vi "AlliGator Batch Dataset Export Window.vi"() -> ()   [LabVIEW 2021, in "AlliGator Files.lvlib"]
doc: "GUI for batch .ptu datasets export to HDF5 files or folders of TIFF images."
uses:
  AlliGator Files.lvlib
  Scripts/AlliGator Data Load & Process Options.ctl
  Scripts/AlliGator Data Information.ctl
  Settings/AlliGator Background Subtraction Parameters.ctl
  Settings/AlliGator Define Gates to.ctl
  Settings/AlliGator Gates to Keep.ctl
  Settings/AlliGator Gate Arithmetic.ctl
  Scripts/AlliGator Source Image Settings.ctl
  Settings/AlliGator Low Count Pixels Rejection Options.ctl
  Settings/AlliGator High Count Pixels Rejection Options.ctl
  Settings/AlliGator Image Smoothing Options.ctl
  Arrays/Kernel Type.ctl
  Arrays/Smoothing Algorithm.ctl
  Source Image/AlliGator Image Binning Options.ctl
  Decay Analysis/Decay Preprocessing/AlliGator Decay Preprocessing Options.ctl
  Decay Analysis/Decay Preprocessing/AlliGator Background Subtraction Parameters.ctl
  Decay Analysis/Decay Preprocessing/AlliGator Baseline Subtraction Method.ctl
  Decay Analysis/Decay Preprocessing/AlliGator Decay Preprocessing Parameters.ctl
  Graphs/XY Graph/XY Graph Plot Shift Parameters.ctl
  Graphs/XY Graph/XY Graph Plot Shift Method.ctl
  Globals, Variables, Constants/AlliGator Variables List.ctl
  AlliGator Batch File Conversion Item.ctl
  AlliGator TIFF Series Options.ctl
  AlliGator Saved TIFF Image Type.ctl
  835454da-008c-4cc5-9e1e-46d3d2ae4ada.vi
  <userlib>/_OpenG.lib/array/array.llb/Filter 1D Array with Scalar (Boolean)__ogtk.vi
  <userlib>/_OpenG.lib/array/array.llb/Delete Elements from 1D Array (Variant)__ogtk.vi
  Variant/Variant to Data/Variant to Boolean.vi
  <vilib>/ErrorRing/Error Ring.xnode
  GUI/GUI.lvlib
  <userlib>/_OpenG.lib/array/array.llb/openg_array.lvlib
  Scripts/AlliGator Scripts.lvlib
  Settings/AlliGator Settings.lvlib
  Arrays/Arrays.lvlib
  Source Image/AlliGator Source Image.lvlib
  Decay Analysis/Decay Preprocessing/AlliGator Decay Preprocessing.lvlib
  Graphs/XY Graph/XY Graph Add-Ons.lvlib
  Notebook/Notebook.lvlib
  Rich Text Box/Rich Text Box.lvlib
  Strings/Strings.lvlib
  Globals, Variables, Constants/AlliGator Globals, Variables & Constants.lvlib
  Variant/Variant to Data/Variant to Data.lvlib
  Sound/Sound.lvlib
  Utilities/Utilities.lvlib
panel:
  out "Conversion Jobs":cluster{"File Path":path, "Exported":bool}[](array[cluster])
  out "Message":string
  out "Animated Busy Icon":bool=TRUE
  in  "Abort":bool
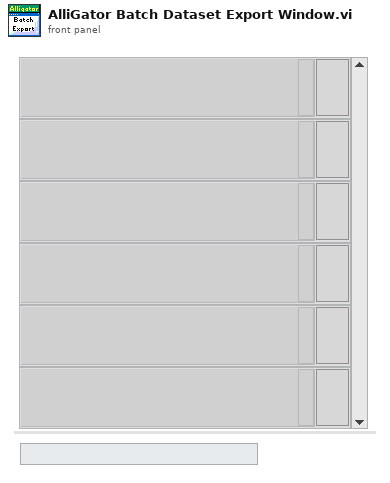
[diagram p1: front panel]
types:
  T1 = typedef "AlliGator Globals, Variables & Constants.lvlib/AlliGator Variables List.ctl" = enum16{"---- GUI ----", "GUI:Initialization Status", "GUI:State Indicators Refnum", "GUI:Original AlliGator Menu Items", "GUI:Current Action Loop State", "GUI:Script in progress", "GUI:Playback", "GUI:Loop Playback", "GUI:Search ROI Used", "GUI:Search ROI", "Decay Graph Max Legend Size", "Intensity Graph Max Legend Size", "Decay Statistics Graph Max Legend Size", "Phasor Graph Max Legend Size", "Phasor Ratio Graph Max Legend Size", "Lifetime Graph Max Legend Size", "---- Files ----", "Files:Export Dataset Frames as Individual Files", "Files:Show Batch Export Help Balloons", "Files:Frames in Dataset", "Files:ptu File Frame Start Indices", "Files:Current Frame in Dataset", "Files:Current Frame Timestamp", "Files:Dataset Loaded", "Files:Dataset Metadata", "Files:Dataset Channel", "Files:Dataset Data Description", "Files:Background Dataset Metadata", "Files:Background Dataset Channel", "Files:Background Dataset Data Description", "Files:Background File Subtraction", "Files:Background File Path", "Files:Background File Pile-up Correction", "Files:Background File Pixel Well Capacity", "Files:Background File Scaling Factor", "Files:Current Dataset Load Settings", "Files:Dataset Path", "Files:ICCD-specific Information", "Files:Macrotime Gate Separation", "------ Python Plugins ------", "Python Plugins:Information", "Python Plugins:Python Session", "Python Plugins:Valid Python Session?", "---- Source Image ----", "Source Image:ROIs", "Source Image:Current ROI", "Source Image:ROI Event Refnum", "X_Source Image Display Range", "X_Source Image Palette Information", "X_Type of Displayed Image", "X_Time Gate Slider", "Source Image:Palette List", "Source Image:Scale", "Source Image:ROI Overlay Color", "Source Image:Overlay to Erase", "Source Image:Is Displayed Image Accumulated", "Source Image:White Light Image Modified", "Source Image:Mask Image Modified", "---- Image Profile Window ----", "Image Profile:Window Event Refnum", "Image Profile:IntensityType", "Image Profile:Intensity Average Type", "Image Profile:Intensity-weighted SDV", "Image Profile:Box Profile Type", "Image Profile:Window Open", "Image Profile:Plotted Fit Parameter", "------ Phasor Graph -------", "Phasor Graph:Show Line", "---- Phasor Plot ---", "Phasor Plot:Parameters Changed", "Phasor Plot:FLI Dataset Modified since last Calculation", "Phasor Harmonics Data", "Selected Phasor Harmonics", "Phasor Harmonic Manager Event Refnum", "Phasor Plot:ROIs", "Phasor Plot:Current ROI", "Phasor Plot:ROI Event Refnum", "Phasor Plot:Image Reference Points", "Phasor Plot:Computed", "Phasor Plot:Palette Information", "Phasor Plot:Palette List", "Phasor Plot:Phasor Ratio Palette Information", "Phasor Plot:Phasor Ratio Palette List", "Phasor Plot:Image Scale", "Phasor Plot:Image Overlay to Erase", "Phasor Plot:Image Elements to Update", "Phasor Plot:Current Calculation Parameters", "Phasor Plot:Current Calibration Options", "Phasor Plot:Reset Cumulated Phasor Plot", "Phasor Plot:Reference 1", "Phasor Plot:Lifetime Reference 1", "Phasor Plot:Reference 1 Frequency", "Phasor Plot:Reference 2", "Phasor Plot:Lifetime Reference 2", "Phasor Plot:Reference 2 Frequency", "---- Decay Analysis ----", "Number of Selected Decays to Fit", "LS Fit Results", "LAR Fit Results", "BS Fit Results", "Last Decay Max - Min", "Best Fit Parameters", "Best Fit Parameter Names", "Actual Size X", "Actual Size Y", "Binning X", "Binning Y", "Actual # Gates", "Dataset Number", "Gates to...", "Gates Skipped", "Gates to keep", "Gate Step", "Gate Separation", "Reversed Gates", "Pile-up Correction", "Pixel Well Capacity", "Background Subtracted", "Background Subtraction Method", "Background Definition Range", "Background File (deprecated)", "Number of Dataset Accumulated", "Array of Accumulated Dataset Paths", "Do Averaged Datasets", "Destination File Path", "Process Plot Target", "Use 1/D as Phasor Frequency", "---- Decay Fit Parameter Map -----", "Decay Fit Parameter Map:Palette Information", "Decay Fit Parameter Map:Palette List", "---- Parameter Map ----", "Parameter Map:Palette Information", "Parameter Map:Palette List", "------- Local Decay Window ---------", "Local Decay Graph Window:Event Refnum", "Local Decay Graph Window:Use normalized IRF for convolution", "----- Miscellaneous ----", "Misc:Skippable Dialog Windows Status"}
  T2 = typedef "AlliGator Scripts.lvlib/AlliGator Data Load & Process Options.ctl" = cluster{"Data Information":T3, "Source Image Settings":T8, "Decay Preprocessing Options & Parameters":T15, "Clear Phasor Graph":bool}
  T3 = typedef "AlliGator Scripts.lvlib/AlliGator Data Information.ctl" = cluster{"Gates to Skip":T4, "# Gates":u32, "Gate Step":u32, "Gate Duration":dbl[unit], "Gate Separation":dbl[unit], "Pile-up Correction":bool, "Pixel Well Capacity":u32, "Define Gates to":T5, "Gates to Keep":T6, "Laser Period":dbl[unit], "SYNC Period":dbl[unit], "Channel Name":u16, "Channel Arithmetic":T7, "Background File Subtraction":bool, "Background Scaling Factor":dbl, "Background File":path, "Background Pile-up Correction":bool, "Background Pixel Well Capacity":u32, "Dataset Scaling Factor":dbl}
  T4 = typedef "AlliGator Settings.lvlib/AlliGator Background Subtraction Parameters.ctl" = cluster{"Start":u32, "End":u32}
  T5 = typedef "AlliGator Settings.lvlib/AlliGator Define Gates to.ctl" = enum32{"Skip", "Keep"}
  T6 = typedef "AlliGator Settings.lvlib/AlliGator Gates to Keep.ctl" = cluster{"First":u32, "Last":u32}
  T7 = typedef "AlliGator Settings.lvlib/AlliGator Gate Arithmetic.ctl" = enum16{"None", "INT-G2", "G2/INT*<INT>", "(1 - G2/INT)*<INT>"}
  T8 = typedef "AlliGator Scripts.lvlib/AlliGator Source Image Settings.ctl" = cluster{"Low Count Pixels Rejection Options":T9, "High Count Pixels Rejection Options":T10, "Peak Threshold":dbl, "Intensity Threshold":dbl, "Image Smoothing Options":T11, "Image Binning Options":T14}
  T9 = typedef "AlliGator Settings.lvlib/AlliGator Low Count Pixels Rejection Options.ctl" = cluster{"Background Low Threshold Factor":dbl, "Fixed Low Background Threshold":dbl, "Reject Low Count Pixels":bool, "Low Percentile":dbl}
  T10 = typedef "AlliGator Settings.lvlib/AlliGator High Count Pixels Rejection Options.ctl" = cluster{"Background High Threshold Factor":dbl, "Fixed High Background Threshold":dbl, "Reject High Count Pixels":bool, "High Percentile":dbl}
  T11 = typedef "AlliGator Settings.lvlib/AlliGator Image Smoothing Options.ctl" = cluster{"Use Image Smoothing":bool, "Kernel Type":T12, "Bin":i32, "Algorithm":T13}
  T12 = typedef "Arrays.lvlib/Kernel Type.ctl" = enum16{"Uniform", "Bilinear", "Gaussian"}
  T13 = typedef "Arrays.lvlib/Smoothing Algorithm.ctl" = enum16{"Rapid", "Thorough"}
  T14 = typedef "AlliGator Source Image.lvlib/AlliGator Image Binning Options.ctl" = cluster{"Use Image Binning":bool, "X Bin":i32, "Y Bin":i32}
  T15 = typedef "AlliGator Decay Preprocessing.lvlib/AlliGator Decay Preprocessing Options.ctl" = cluster{"Background Subtraction Parameters":T16, "Decay Preprocessing Parameters":T18, "Preprocessing Steps Order":string[]}
  T16 = typedef "AlliGator Decay Preprocessing.lvlib/AlliGator Background Subtraction Parameters.ctl" = cluster{"Background Definition Range":cluster{"Min Gate":dbl[unit], "Max Gate":dbl[unit]}, "Baseline Subtraction Method":T17, "Background Subtraction?":bool, "Background File":path, "Background Constant":dbl, "Background Scaling Factor":dbl, "Background Pile-up Correction":bool, "Background Pixel Well Capacity":u32}
  T17 = typedef "AlliGator Decay Preprocessing.lvlib/AlliGator Baseline Subtraction Method.ctl" = enum16{"Mean", "Min", "Square Gated Single-Exponential", "File", "Constant"}
  T18 = typedef "AlliGator Decay Preprocessing.lvlib/AlliGator Decay Preprocessing Parameters.ctl" = cluster{"Background Subtraction":bool, "Straighten Decay":bool, "Reverse Gates":bool, "1-Normalized Decay":bool, "Smoothen Decay":bool, "Smoothing Parameter":dbl, "Shift Decay":bool, "Decay Shift Parameters":T19, "Extrapolate Decay":bool, "Additional Points":u32, "Head Fraction":dbl, "Pixel-Normalize Decay":bool, "Use Periodicity":bool, "Use Cursors":bool, "Tail Fraction":dbl, "Use Decay Pre-Processing":bool, "Fold Decay":bool, "# Folds":u32, "[0-1]-Normalized Decay":bool}
  T19 = typedef "XY Graph Add-Ons.lvlib/XY Graph Plot Shift Parameters.ctl" = cluster{"Type":T20, "Shift":dbl[unit], "Threshold":dbl, "Rotate":bool}
  T20 = typedef "XY Graph Add-Ons.lvlib/XY Graph Plot Shift Method.ctl" = enum16{"Default", "CFD", "Threshold", "Cross-Correlation"}
  T21 = typedef "AlliGator Files.lvlib/AlliGator Batch File Conversion Item.ctl" = cluster{"File Path":path, "Saved":bool}
  T22 = typedef "AlliGator Files.lvlib/AlliGator Saved TIFF Image Type.ctl" = enum16{"Single Gate", "Sum of All Gates", "Phasor"}
  T23 = typedef "AlliGator Files.lvlib/AlliGator TIFF Series Options.ctl" = cluster{"Gate Image File Name":string, "File Number Format":string, "Start Index":u32, "Save Metadata File":bool, "Compress Image":bool}
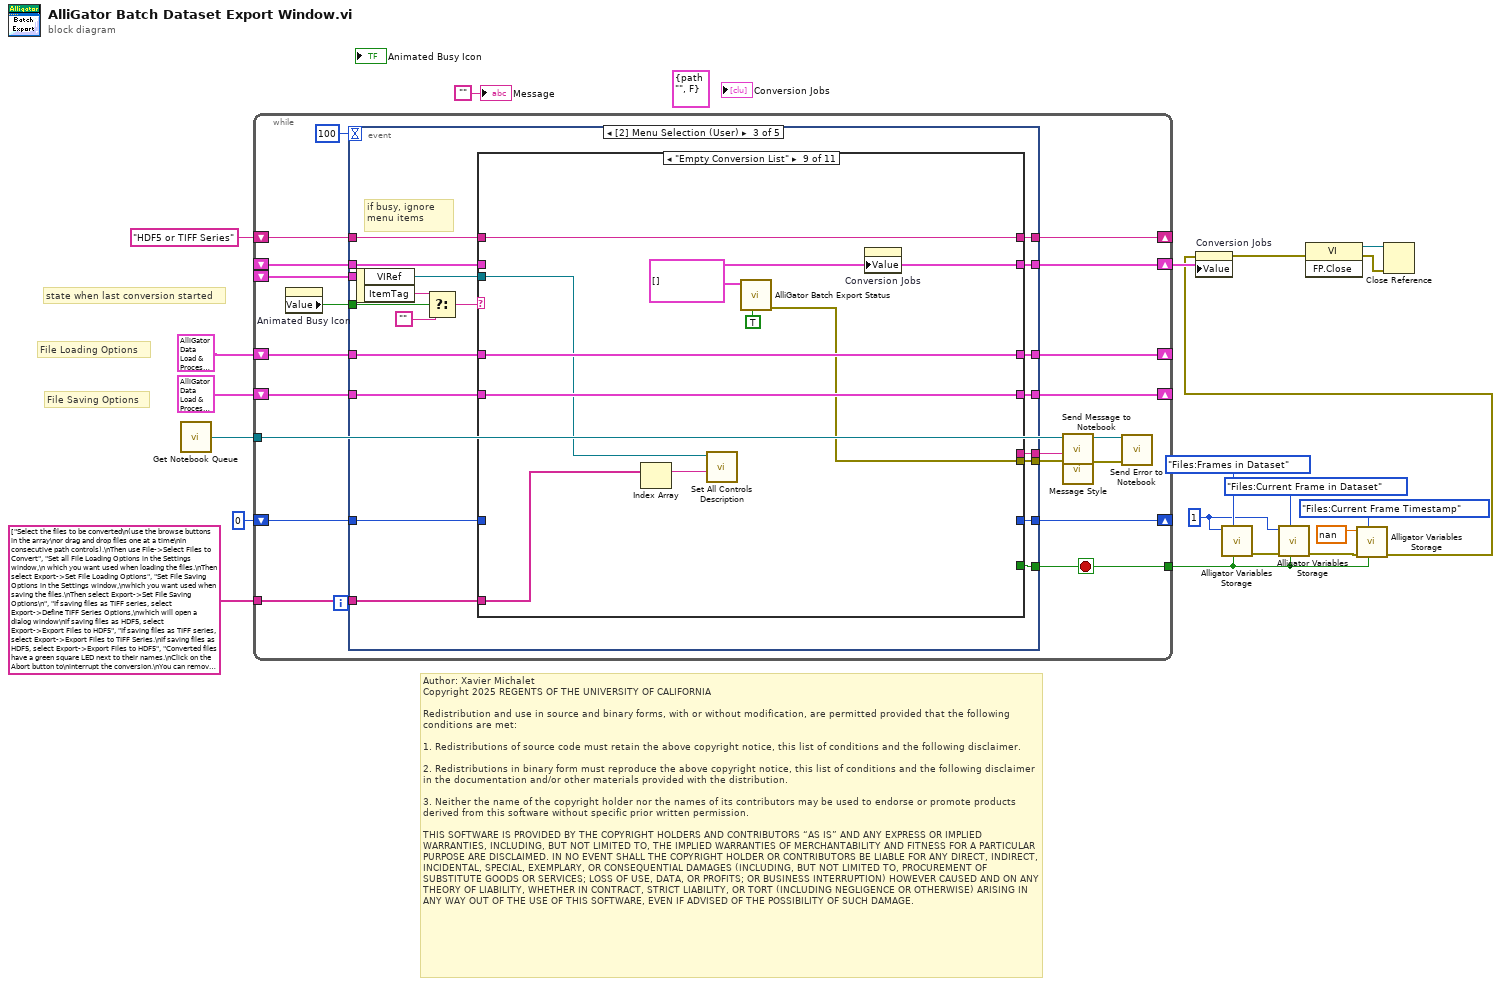
[diagram p0: block diagram]
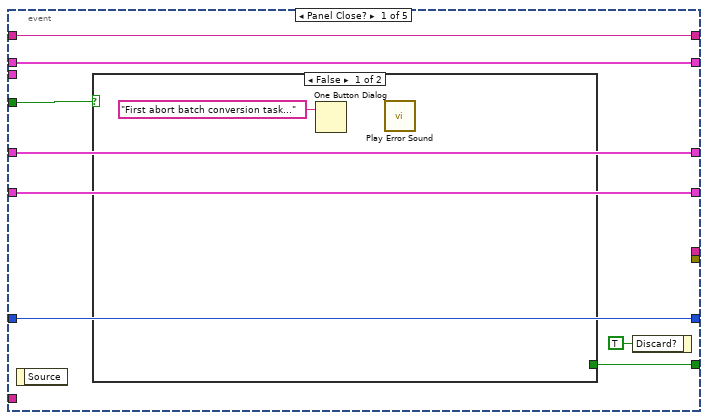
[diagram p2: hidden frame]
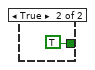
[diagram p3: hidden frame]
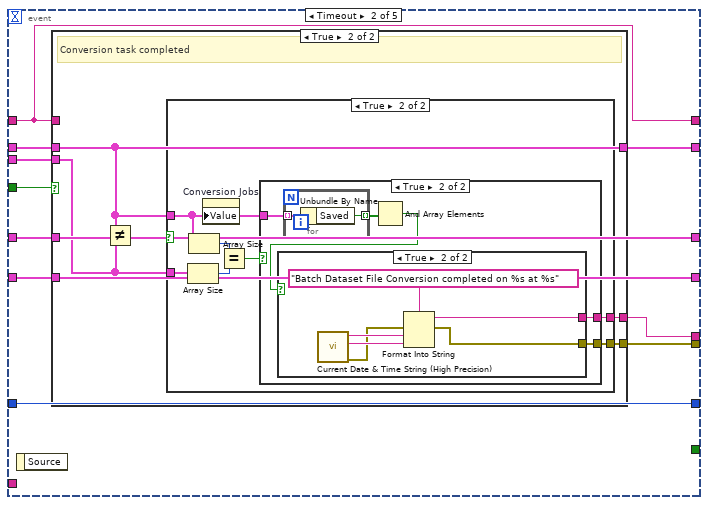
[diagram p4: hidden frame]
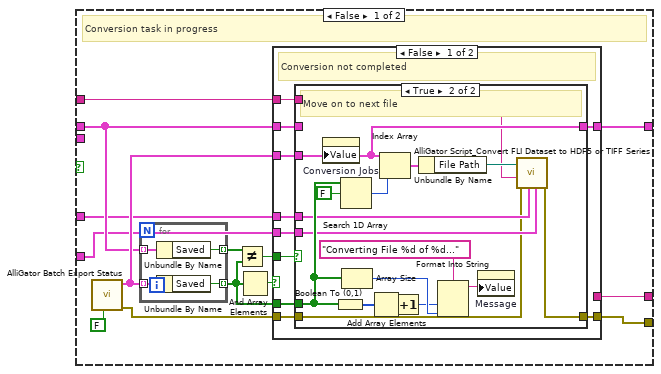
[diagram p5: hidden frame]
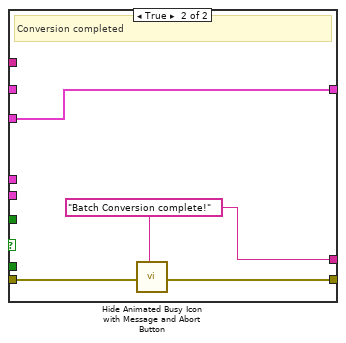
[diagram p7: hidden frame]
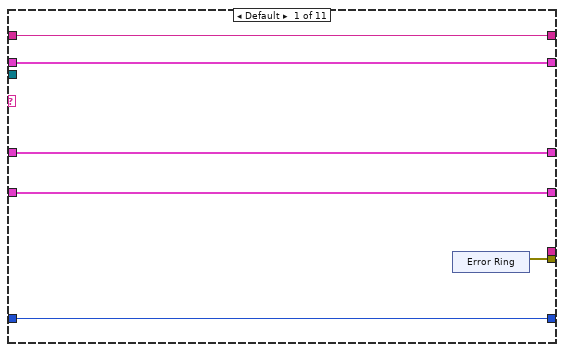
[diagram p11: hidden frame]
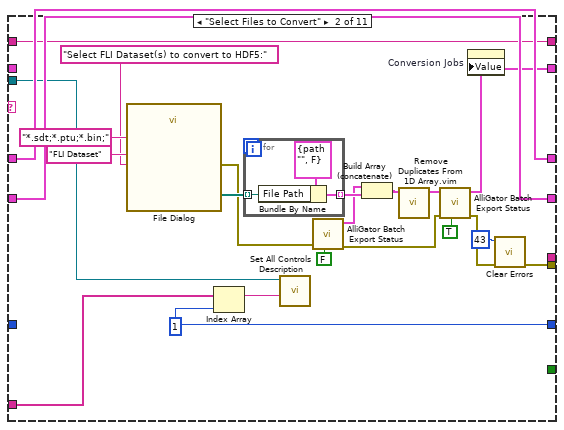
[diagram p12: hidden frame]
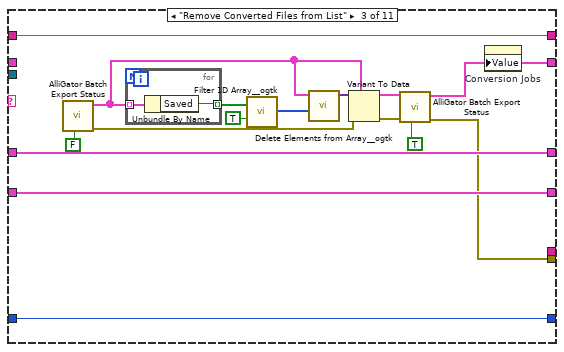
[diagram p13: hidden frame]
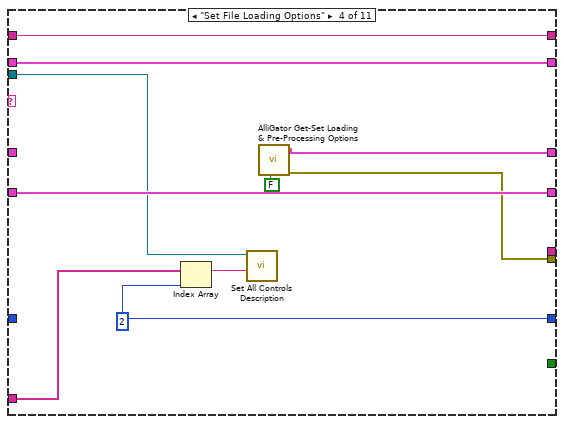
[diagram p14: hidden frame]
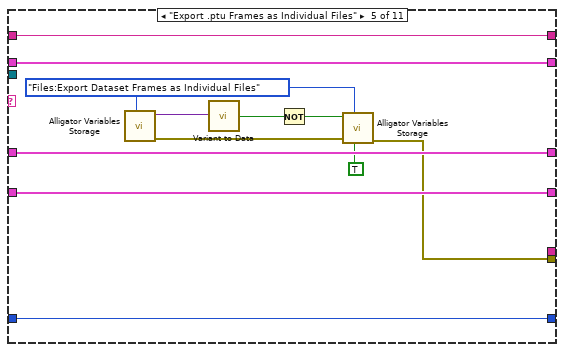
[diagram p15: hidden frame]
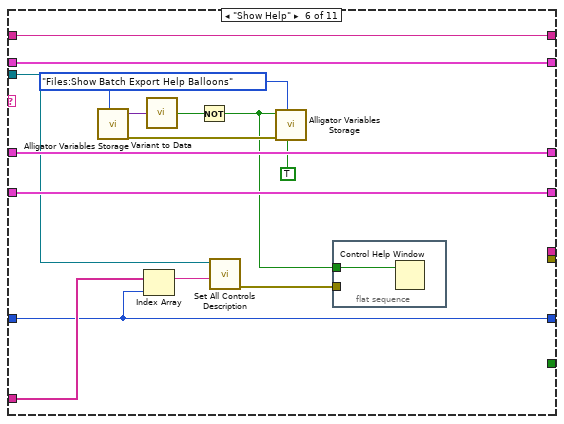
[diagram p16: hidden frame]
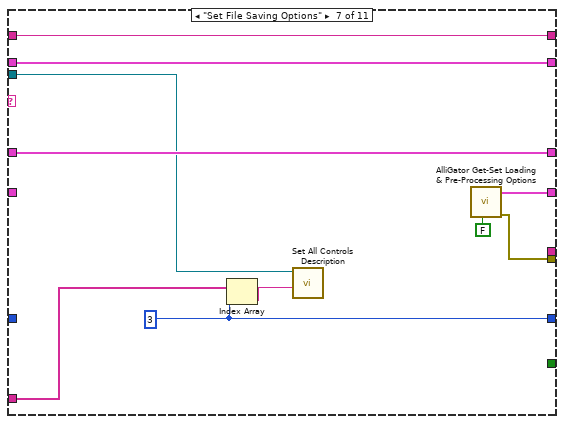
[diagram p17: hidden frame]
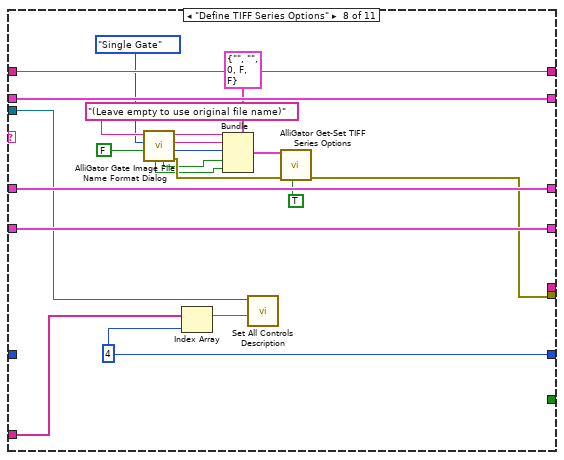
[diagram p18: hidden frame]
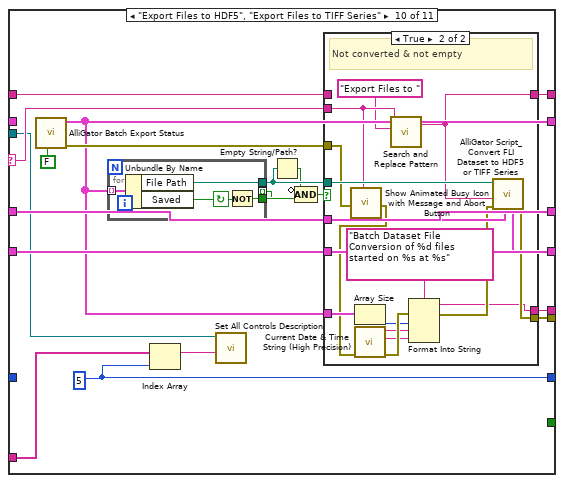
[diagram p19: hidden frame]
diagram:
  w8 = 1
  (unwired) T21 {"File Path"=path "", "Saved"=FALSE} ("File Array")
  # "Author: Xavier Michalet\nCopyright 2025 REGENTS OF THE UNIVERSITY OF CALIFORNIA\n\nRedistribution and use in source and binary forms, with or without modification, are permitted provided that the following conditions are met:\n\n1. Redistributions of source code must retain the above copyright notice, this list of conditions and the following disclaimer.\n\n2. Redistributions in binary form must reproduce the above copyright notice, this list of conditions and the following disclaimer in the documentation and/or other materials provided with the distribution.\n\n3. Neither the name of the copyright holder nor the names of its contributors may be used to endorse or promote products derived from this software without specific prior written permission.\n\nTHIS SOFTWARE IS PROVIDED BY THE COPYRIGHT HOLDERS AND CONTRIBUTORS “AS IS” AND ANY EXPRESS OR IMPLIED WARRANTIES, INCLUDING, BUT NOT LIMITED TO, THE IMPLIED WARRANTIES OF MERCHANTABILITY AND FITNESS FOR A PARTICULAR PURPOSE ARE DISCLAIMED. IN NO EVENT SHALL THE COPYRIGHT HOLDER OR CONTRIBUTORS BE LIABLE FOR ANY DIRECT, INDIRECT, INCIDENTAL, SPECIAL, EXEMPLARY, OR CONSEQUENTIAL DAMAGES (INCLUDING, BUT NOT LIMITED TO, PROCUREMENT OF SUBSTITUTE GOODS OR SERVICES; LOSS OF USE, DATA, OR PROFITS; OR BUSINESS INTERRUPTION) HOWEVER CAUSED AND ON ANY THEORY OF LIABILITY, WHETHER IN CONTRACT, STRICT LIABILITY, OR TORT (INCLUDING NEGLIGENCE OR OTHERWISE) ARISING IN ANY WAY OUT OF THE USE OF THIS SOFTWARE, EVEN IF ADVISED OF THE POSSIBILITY OF SUCH DAMAGE."
  # "File Saving Options"
  # "File Loading Options"
  # "state when last conversion started"
  n1 = call "Get Notebook Queue.vi"() -> ("Notebook Queue"=w3:refnum<queue>)  [unwired: 9 in]
  n2 = while {
    shift-right: [w39] -> w19
    shift-left: _ -> [w37]
    shift-left: _ -> [w38]
    shift-right: [w36] -> _
    shift-left: T2 {"Data Information"={"Gates to Skip"={"Start"=0, "End"=0}, "# Gates"=1, "Gate Step"=1, "Gate Duration"=3e-10, "Gate Separation"=4e-11, "Pile-up Correction"=FALSE, "Pixel Well Capacity"=1, "Define Gates to"=enum."Skip", "Gates to Keep"={"First"=0, "Last"=0}, "Laser Period"=0.0, "SYNC Period"=0.0, "Channel Name"=0, "Channel Arithmetic"=enum."None", "Background File Subtraction"=FALSE, "Background Scaling Factor"=1.0, "Background File"=path "", "Background Pile-up Correction"=FALSE, "Background Pixel Well Capacity"=1, "Dataset Scaling Factor"=1.0}, "Source Image Settings"={"Low Count Pixels Rejection Options"={"Background Low Threshold Factor"=0.0, "Fixed Low Background Threshold"=20000.0, "Reject Low Count Pixels"=FALSE, "Low Percentile"=0.0}, "High Count Pixels Rejection Options"={"Background High Threshold Factor"=0.0, "Fixed High Background Threshold"=1.0, "Reject High Count Pixels"=FALSE, "High Percentile"=100.0}, "Peak Threshold"=500.0, "Intensity Threshold"=500.0, "Image Smoothing Options"={"Use Image Smoothing"=FALSE, "Kernel Type"=enum."Bilinear", "Bin"=1, "Algorithm"=enum."Rapid"}, "Image Binning Options"={"Use Image Binning"=FALSE, "X Bin"=1, "Y Bin"=1}}, "Decay Preprocessing Options & Parameters"={"Background Subtraction Parameters"={"Background Definition Range"={"Min Gate"=0.0, "Max Gate"=0.0}, "Baseline Subtraction Method"=enum."Mean", "Background Subtraction?"=FALSE, "Background File"=path "", "Background Constant"=0.0, "Background Scaling Factor"=1.0, "Background Pile-up Correction"=FALSE, "Background Pixel Well Capacity"=1}, "Decay Preprocessing Parameters"={"Background Subtraction"=FALSE, "Straighten Decay"=FALSE, "Reverse Gates"=FALSE, "1-Normalized Decay"=FALSE, "Smoothen Decay"=FALSE, "Smoothing Parameter"=0.0, "Shift Decay"=FALSE, "Decay Shift Parameters"={"Type"=enum."Default", "Shift"=0.0, "Threshold"=0.0, "Rotate"=FALSE}, "Extrapolate Decay"=FALSE, "Additional Points"=0, "Head Fraction"=0.0, "Pixel-Normalize Decay"=FALSE, "Use Periodicity"=FALSE, "Use Cursors"=FALSE, "Tail Fraction"=0.0, "Use Decay Pre-Processing"=TRUE, "Fold Decay"=FALSE, "# Folds"=1, "[0-1]-Normalized Decay"=FALSE}, "Preprocessing Steps Order"=[]}, "Clear Phasor Graph"=FALSE} ("Dataset Loading & Pre-processing Options (out)") -> [w35]
    shift-right: [w34] -> _
    shift-left: T2 {"Data Information"={"Gates to Skip"={"Start"=0, "End"=0}, "# Gates"=1, "Gate Step"=1, "Gate Duration"=3e-10, "Gate Separation"=4e-11, "Pile-up Correction"=FALSE, "Pixel Well Capacity"=1, "Define Gates to"=enum."Skip", "Gates to Keep"={"First"=0, "Last"=0}, "Laser Period"=0.0, "SYNC Period"=0.0, "Channel Name"=0, "Channel Arithmetic"=enum."None", "Background File Subtraction"=FALSE, "Background Scaling Factor"=1.0, "Background File"=path "", "Background Pile-up Correction"=FALSE, "Background Pixel Well Capacity"=1, "Dataset Scaling Factor"=1.0}, "Source Image Settings"={"Low Count Pixels Rejection Options"={"Background Low Threshold Factor"=0.0, "Fixed Low Background Threshold"=20000.0, "Reject Low Count Pixels"=FALSE, "Low Percentile"=0.0}, "High Count Pixels Rejection Options"={"Background High Threshold Factor"=0.0, "Fixed High Background Threshold"=1.0, "Reject High Count Pixels"=FALSE, "High Percentile"=100.0}, "Peak Threshold"=500.0, "Intensity Threshold"=500.0, "Image Smoothing Options"={"Use Image Smoothing"=FALSE, "Kernel Type"=enum."Bilinear", "Bin"=1, "Algorithm"=enum."Rapid"}, "Image Binning Options"={"Use Image Binning"=FALSE, "X Bin"=1, "Y Bin"=1}}, "Decay Preprocessing Options & Parameters"={"Background Subtraction Parameters"={"Background Definition Range"={"Min Gate"=0.0, "Max Gate"=0.0}, "Baseline Subtraction Method"=enum."Mean", "Background Subtraction?"=FALSE, "Background File"=path "", "Background Constant"=0.0, "Background Scaling Factor"=1.0, "Background Pile-up Correction"=FALSE, "Background Pixel Well Capacity"=1}, "Decay Preprocessing Parameters"={"Background Subtraction"=FALSE, "Straighten Decay"=FALSE, "Reverse Gates"=FALSE, "1-Normalized Decay"=FALSE, "Smoothen Decay"=FALSE, "Smoothing Parameter"=0.0, "Shift Decay"=FALSE, "Decay Shift Parameters"={"Type"=enum."Default", "Shift"=0.0, "Threshold"=0.0, "Rotate"=FALSE}, "Extrapolate Decay"=FALSE, "Additional Points"=0, "Head Fraction"=0.0, "Pixel-Normalize Decay"=FALSE, "Use Periodicity"=FALSE, "Use Cursors"=FALSE, "Tail Fraction"=0.0, "Use Decay Pre-Processing"=TRUE, "Fold Decay"=FALSE, "# Folds"=1, "[0-1]-Normalized Decay"=FALSE}, "Preprocessing Steps Order"=[]}, "Clear Phasor Graph"=FALSE} ("Dataset Loading & Pre-processing Options (out)") -> [w33]
    tunnel: w3 -> [w28]
    shift-right: [w32] -> _
    shift-left: "HDF5 or TIFF Series" ("result string") -> [w31]
    tunnel: string[] ["Select the files to be converted\n(use the browse buttons in the array\nor drag and drop files one at a time\nin consecutive path controls).\nThen use File->Select Files to Convert", "Set all File Loading Options in the Settings window,\n which you want used when loading the files.\nThen select Export->Set File Loading Options", "Set File Saving Options in the Settings window,\nwhich you want used when saving the files.\nThen select Export->Set File Saving Options\n", "If saving files as TIFF series, select Export->Define TIFF Series Options,\nwhich will open a dialog window\nIf saving files as HDF5, select Export->Export Files to HDF5", "If saving files as TIFF series, select Export->Export Files to TIFF Series.\nIf saving files as HDF5, select Export->Export Files to HDF5", "Converted files have a green square LED next to their names.\nClick on the Abort button to\ninterrupt the conversion.\nYou can remove the converted files\nfrom the list using File->Remove Converted Files from List."] ("Text") -> [w29]
    shift-right: [w23] -> _
    shift-left: 0 ("index") -> [w22]
    tunnel: [w21] -> w1
    stop <- w21 stop-if-true
    n3 = property on="Animated Busy Icon" class="Bool (strict)"() -> ("Value"=w30:bool)  [unwired: 2 in, 2 out]
    n4 = event shown="[2] Menu Selection (User)" {
      selector: _ -> [_ _ _ _ _]
      dyn-events: _ -> [_ _ _ _ _]
      timeout: 100 -> [_ _ _ _ _]
      tunnel: w30 -> [w48 w60 w155 _ _]
      tunnel: [w46 _ w153 _ _] -> w21
      tunnel: [w45 w58 w152 w343 w364] -> w39
      tunnel: w38 -> [w45 w59 w151 w343 w364]
      tunnel: w37 -> [_ w57 _ _ _]
      tunnel: [w44 w56 w148 w352 w363] -> w36
      tunnel: w35 -> [w44 w56 w147 w352 w363]
      tunnel: [w43 w55 w146 w351 w362] -> w34
      tunnel: w33 -> [w43 w55 w145 w351 w362]
      tunnel: [_ w54 w144 _ w360] -> w25
      tunnel: [w42 w53 w143 w350 w361] -> w32
      tunnel: w31 -> [w42 w53 w142 w350 w361]
      tunnel: w29 -> [_ _ w141 _ _]
      tunnel: [_ w52 w140 _ w354] -> w26
      tunnel: [w41 w51 w138 w337 w353] -> w23
      tunnel: w22 -> [w41 w51 w137 w337 w353]
      event Panel Close? {
        n5 = event-data() -> ()  [unwired: 1 in, 1 out]
        n6 = case shown="False" w48 {
          tunnel: [_ TRUE ("Discard?")] -> w46
          frame False {
            n7 = One Button Dialog(message="First abort batch conversion task...") -> ()  [unwired: 1 in, 1 out]
            n8 = call "Play Error Sound.vi"() -> ()  [unwired: 27 in, 1 out]
          }
          frame True {
          }
        }
        n9 = event-data("Discard?"=TRUE) -> ()  [unwired: 1 in, 1 out]
      }
      event Timeout {
        n10 = event-data() -> ()  [unwired: 1 in, 1 out]
        n11 = case shown="True" w60 {
          tunnel: w59 -> [w69 w115]
          tunnel: [w71 w115] -> w58
          tunnel: w57 -> [_ w113]
          tunnel: w56 -> [w65 _]
          tunnel: w55 -> [w64 _]
          tunnel: [w63 w114] -> w54
          tunnel: w53 -> [w62 _]
          tunnel: [w61 w112] -> w52
          frame False {
            # "Conversion task in progress"
            n12 = call "AlliGator Batch Export Status.vi"("Set/Get (F)"=FALSE) -> ("error out"=w72:errorcluster, "Conversion Jobs out"=w70:T21[])  [unwired: 9 in]
            n13 = for {
              tunnel: w70 -> [w78] mode=indexing
              tunnel: [w77] -> w67 mode=indexing
              tunnel: w69 -> [w76] mode=indexing
              tunnel: [w75] -> w68 mode=indexing
              n14 = Unbundle By Name(w76) -> ("Saved"=w75:bool)
              n15 = Unbundle By Name(w78) -> ("Saved"=w77:bool)
            }
            n16 = Not Equal?(x=w68, y=w67) -> (x != y?=w66:bool)
            n17 = And Array Elements(Boolean array=w67) -> (logical AND=w73:bool)
            n18 = case shown="False" w73 {
              tunnel: w67 -> [w88 _]
              tunnel: w72 -> [w81 w111]
              tunnel: [w85 w110] -> w71
              tunnel: w70 -> [w84 w110]
              tunnel: w69 -> [w86 _]
              tunnel: w66 -> [w87 _]
              tunnel: w65 -> [w83 _]
              tunnel: w64 -> [w82 _]
              tunnel: [w80 w109] -> w63
              tunnel: w62 -> [w79 _]
              tunnel: [_ w108] -> w61
              frame False {
                # "Conversion not completed"
                n19 = case shown="True" w87 {
                  tunnel: w88 -> [_ w101]
                  tunnel: w86 -> [w90 _]
                  tunnel: [w90 w96] -> w85
                  tunnel: w84 -> [_ w96]
                  tunnel: w83 -> [_ w95]
                  tunnel: w82 -> [_ w94]
                  tunnel: w81 -> [w89 w93]
                  tunnel: [w89 w92] -> w80
                  tunnel: w79 -> [_ w91]
                  frame False {
                    # "conversion not complete"
                  }
                  frame True {
                    # "Move on to next file"
                    n20 = property on="Conversion Jobs" class="Arr"("Value"=w96) -> ()  [unwired: 2 in, 2 out]
                    n21 = Boolean To (0,1)(Boolean=w101) -> (0, 1=w107:i16[])
                    n22 = Search 1D Array(1D array=w101, element=FALSE) -> (index of element=w99:i32)  [unwired: 1 in]
                    n23 = Array Size(array=w101) -> (size(s)=w105:i32)
                    n24 = Add Array Elements(numeric array=w107) -> (sum=w106:i16)
                    n25 = Index Array(array=w96, index=w99) -> (element=w98:T21)
                    n26 = Increment(x=w106) -> (x+1=w102:i16)
                    n27 = Unbundle By Name(w98) -> ("File Path"=w97:path)
                    n28 = Format Into String(format string="Converting File %d of %d...", w102, w105) -> (resulting string=w103:string)  [unwired: 2 in, 1 out]
                    n29 = property on="Message" class="Str"("Value"=w103) -> ()  [unwired: 2 in, 2 out]
                    n30 = call "AlliGator Script_Convert FLI Dataset to HDF5 or TIFF Series.vi"("Dataset Saving Options"=w94, "Dataset Loading Options"=w95, "Error In"=w93, "Destination File Type"=w91, "File Path"=w97) -> ("Error Out"=w92:errorcluster)  [unwired: 6 in]
                  }
                }
              }
              frame True {
                w108 = "Batch Conversion complete!" ("Message")
                # "Conversion completed"
                n31 = call "Hide Animated Busy Icon with Message and Abort Button.vi"("Message"=w108, "Error In"=w111) -> ("Error Out"=w109:errorcluster)  [unwired: 17 in]
              }
            }
          }
          frame True {
            # "Conversion task completed"
            n32 = Not Equal?(x=w115, y=w113) -> (x != y?=w116:bool)
            n33 = case shown="True" w116 {
              tunnel: w115 -> [_ w118]
              tunnel: [_ w123] -> w114
              tunnel: w113 -> [_ w122]
              tunnel: [_ w117] -> w112
              frame False {
              }
              frame True {
                n34 = Array Size(array=w122) -> (size(s)=w120:i32)
                n35 = Array Size(array=w118) -> (size(s)=w121:i32)
                n36 = property on="Conversion Jobs" class="Arr"("Value"=w118) -> ()  [unwired: 2 in, 2 out]
                n37 = Equal?(x=w121, y=w120) -> (x = y?=w119:bool)
                n38 = case shown="True" w119 {
                  tunnel: [_ w128] -> w123
                  tunnel: w118 -> [_ w127]
                  tunnel: [_ w124] -> w117
                  frame False {
                  }
                  frame True {
                    n39 = for {
                      tunnel: w127 -> [w136] mode=indexing
                      tunnel: [w135] -> w126 mode=indexing
                      n40 = Unbundle By Name(w136) -> ("Saved"=w135:bool)
                    }
                    n41 = And Array Elements(Boolean array=w126) -> (logical AND=w125:bool)
                    n42 = case shown="True" w125 {
                      tunnel: [_ w130] -> w128
                      tunnel: [_ w129] -> w124
                      frame False {
                      }
                      frame True {
                        n43 = call "Current Date & Time String (High Precision).vi"() -> ("Error Out"=w132:errorcluster, "time string"=w133:string, "date string"=w134:string)  [unwired: 8 in, 1 out]
                        n44 = Format Into String(format string="Batch Dataset File Conversion completed on %s at %s", error in=w132, w134, w133) -> (resulting string=w129:string, error out=w130:errorcluster)  [unwired: 1 in]
                      }
                    }
                  }
                }
              }
            }
          }
        }
      }
      event Menu Selection (User) {
        # "if busy, ignore menu items"
        n45 = event-data() -> ("VIRef"=w139:refnum<vi>, "ItemTag"=w150:string)  [unwired: 1 in]
        n46 = Select(t=w150, s=w155, f="") -> (s? t:f=w154:string)
        n47 = case shown="\"Empty Conversion List\"" w154 {
          selector: w154 -> [_ _ _ _ _ _ _ _ _ w292 _]
          tunnel: [_ _ _ _ _ _ _ _ _ _ TRUE] -> w153
          tunnel: [w161 w167 w190 w214 w228 w243 w253 w275 w283 w293 w333] -> w152
          tunnel: w151 -> [w161 _ _ w214 w228 w243 w253 w275 _ _ w333]
          tunnel: [w160 w180 w194 w215 w227 w242 w251 w274 w282 w296 w332] -> w148
          tunnel: w147 -> [w160 w180 w194 _ w227 w242 w251 w274 w282 w296 w332]
          tunnel: [w159 w181 w193 w213 w226 w241 w252 w273 w281 w295 w331] -> w146
          tunnel: w145 -> [w159 w181 w193 w213 w226 w241 _ w273 w281 w295 w331]
          tunnel: [w157 w169 w192 w212 w218 _ w250 w259 w280 w294 w329] -> w144
          tunnel: [w158 w177 w191 w211 w225 w240 w249 w261 w279 w291 w330] -> w143
          tunnel: w142 -> [w158 w177 w191 w211 w225 w240 w249 w261 w279 w290 w330]
          tunnel: w141 -> [_ w166 _ w210 _ w239 w248 w258 w277 w288 w328]
          tunnel: [_ _ _ _ _ _ _ _ _ w289 _] -> w140
          tunnel: w139 -> [_ w163 _ w207 _ w236 w245 w255 w278 w285 w326]
          tunnel: [w156 w165 w189 w209 w217 w237 w247 w257 _ w287 _] -> w138
          tunnel: w137 -> [w156 _ w189 _ w217 w237 _ _ _ _ _]
          frame Default {
            n48 = xnode "Error Ring"() -> ("error out"=w157:errorcluster)
          }
          frame "Select Files to Convert" {
            w165 = 1 ("index")
            n49 = call "File Dialog"("prompt"="Select FLI Dataset(s) to convert to HDF5:", "pattern (all files)"="*.sdt;*.ptu;*.bin;", "pattern label"="FLI Dataset") -> ("selected paths"=w182:path[], "error out"=w179:errorcluster)  [unwired: 9 in, 2 out]
            n50 = Index Array(array=w166, index=w165) -> (element=w164:string)
            n51 = for {
              tunnel: w182 -> [w187] mode=indexing
              tunnel: [w188] -> w176 mode=indexing
              n52 = Bundle By Name(cluster=T21 {"File Path"=path "", "Saved"=FALSE} ("File Array"), "File Path"=w187) -> (w188:T21)
            }
            n53 = call "Set All Controls Description.vi"("Description"=w164, "VI Ref"=w163) -> ()  [unwired: 9 in, 1 out]
            n54 = call "AlliGator Batch Export Status.vi"("Set/Get (F)"=FALSE, "error in (no error)"=w179) -> ("error out"=w170:errorcluster, "Conversion Jobs out"=w174:T21[])  [unwired: 8 in]
            n55 = Build Array (concatenate)(w174, w176) -> (w175:T21[])
            n56 = call "Remove Duplicates From 1D Array.vim"("array"=w175) -> ("array with duplicates removed"=w172:T21[])  [unwired: 10 in]
            n57 = call "AlliGator Batch Export Status.vi"("Set/Get (F)"=TRUE, "error in (no error)"=w170, "Conversion Jobs in"=w172) -> ("error out"=w178:errorcluster, "Conversion Jobs out"=w167:T21[])  [unwired: 7 in]
            n58 = property on="Conversion Jobs" class="Arr"("Value"=w167) -> ()  [unwired: 2 in, 2 out]
            n59 = call <vilib>:"Clear Errors.vi"("error in (no error)"=w178, "specific error code to clear (0: all)"=43) -> ("error out"=w169:errorcluster)  [unwired: 4 in, 1 out]
          }
          frame "Remove Converted Files from List" {
            n60 = call "AlliGator Batch Export Status.vi"("Set/Get (F)"=FALSE) -> ("error out"=w195:errorcluster, "Conversion Jobs out"=w198:T21[])  [unwired: 9 in]
            n61 = for {
              tunnel: w198 -> [w206] mode=indexing
              tunnel: [w205] -> w204 mode=indexing
              n62 = Unbundle By Name(w206) -> ("Saved"=w205:bool)
            }
            n63 = call-poly <userlib>:"Filter 1D Array__ogtk.vi"("items to filter"=TRUE ("Boolean"), "array"=w204) -> ("filtered item indices"=w202:i32[])  [unwired: 4 in, 1 out]
            n64 = call-poly <userlib>:"Delete Elements from Array__ogtk.vi"("indices"=w202, "array"=w198) -> ("array w/ subset deleted"=w200:variant[])  [unwired: 8 in, 1 out]
            n65 = Variant To Data(error in=w195, type=w198, Variant=w200) -> (data=w199:T21[], error out=w196:errorcluster)
            n66 = call "AlliGator Batch Export Status.vi"("Set/Get (F)"=TRUE, "error in (no error)"=w196, "Conversion Jobs in"=w199) -> ("error out"=w192:errorcluster, "Conversion Jobs out"=w190:T21[])  [unwired: 7 in]
            n67 = property on="Conversion Jobs" class="Arr"("Value"=w190) -> ()  [unwired: 2 in, 2 out]
          }
          frame "Set File Loading Options" {
            w209 = 2 ("index")
            n68 = Index Array(array=w210, index=w209) -> (element=w208:string)
            n69 = call "Set All Controls Description.vi"("Description"=w208, "VI Ref"=w207) -> ()  [unwired: 9 in, 1 out]
            n70 = call "AlliGator Get-Set Loading & Pre-Processing Options.vi"("Get (F)/Set"=FALSE) -> ("Error Out"=w212:errorcluster, "Dataset Loading & Pre-processing Options (out)"=w215:T2)  [unwired: 9 in]
          }
          frame "Export .ptu Frames as Individual Files" {
            w224 = AlliGator_Variables_List."Files:Export Dataset Frames as Individual Files" ("Alligator Variable")
            n71 = call "Alligator Variables Storage.vi"("AlliGator Variable"=w224) -> ("Error Out"=w223:errorcluster, "Data out"=w222:variant)  [unwired: 8 in, 1 out]
            n72 = call-poly "Variant to Data.vi"("Variant"=w222) -> ("Value"=w221:bool)  [unwired: 8 in]
            n73 = Not(x=w221) -> (.not. x?=w220:bool)
            n74 = call "Alligator Variables Storage.vi"("Get(F)/Set"=TRUE, "AlliGator Variable"=w224, "Error In"=w223, "Data in"=w220) -> ("Error Out"=w218:errorcluster)  [unwired: 5 in, 2 out]
          }
          frame "Show Help" {
            w231 = AlliGator_Variables_List."Files:Show Batch Export Help Balloons" ("Alligator Variable")
            n75 = call "Alligator Variables Storage.vi"("AlliGator Variable"=w231) -> ("Error Out"=w232:errorcluster, "Data out"=w234:variant)  [unwired: 8 in, 1 out]
            n76 = Index Array(array=w239, index=w237) -> (element=w238:string)
            n77 = call-poly "Variant to Data.vi"("Variant"=w234) -> ("Value"=w233:bool)  [unwired: 8 in]
            n78 = Not(x=w233) -> (.not. x?=w229:bool)
            n79 = call "Set All Controls Description.vi"("Description"=w238, "VI Ref"=w236) -> ("Error Out"=w235:errorcluster)  [unwired: 9 in]
            n80 = call "Alligator Variables Storage.vi"("Get(F)/Set"=TRUE, "AlliGator Variable"=w231, "Error In"=w232, "Data in"=w229) -> ()  [unwired: 5 in, 3 out]
            n81 = flat-sequence {
              tunnel: w235 -> [_]
              tunnel: w229 -> [w244]
              frame #0 {
                n82 = Control Help Window(1:w244) -> ()  [unwired: 1 in]
              }
            }
          }
          frame "Set File Saving Options" {
            w247 = 3 ("index")
            n83 = Index Array(array=w248, index=w247) -> (element=w246:string)
            n84 = call "Set All Controls Description.vi"("Description"=w246, "VI Ref"=w245) -> ()  [unwired: 9 in, 1 out]
            n85 = call "AlliGator Get-Set Loading & Pre-Processing Options.vi"("Get (F)/Set"=FALSE) -> ("Error Out"=w250:errorcluster, "Dataset Loading & Pre-processing Options (out)"=w252:T2)  [unwired: 9 in]
          }
          frame "Define TIFF Series Options" {
            w257 = 4 ("index")
            n86 = call "AlliGator Gate Image File Name Format Dialog.vi"("Single Image"=FALSE, "Saved TIFF Image"=AlliGator_Saved_TIFF_Image_Type."Single Gate", "Image File Name in"="(Leave empty to use original file name)") -> ("error out"=w268:errorcluster, "Start Index out"=w266:u32, "File Number Format out"=w269:string, "Gate Image File Name out"=w270:string, "Compress Image out"=w265:bool, "Save Metadata File out"=w264:bool)  [unwired: 2 in, 1 out]
            n87 = Index Array(array=w258, index=w257) -> (element=w256:string)
            n88 = Bundle(cluster=T23 {"Gate Image File Name"="", "File Number Format"="", "Start Index"=0, "Save Metadata File"=FALSE, "Compress Image"=FALSE} ("output cluster"), "Gate Image File Name"=w270, "File Number Format"=w269, "Start Index"=w266, "Save Metadata File"=w265, "Compress Image"=w264) -> (w263:T23)
            n89 = call "Set All Controls Description.vi"("Description"=w256, "VI Ref"=w255) -> ()  [unwired: 9 in, 1 out]
            n90 = call "AlliGator Get-Set TIFF Series Options.vi"("Set/Get (F)"=TRUE, "error in (no error)"=w268, "output cluster in"=w263) -> ("error out"=w259:errorcluster)  [unwired: 7 in, 1 out]
          }
          frame "Empty Conversion List" {
            w283 = T21[] [] ("Conversion Jobs in")
            n91 = Index Array(array=w277) -> (element=w276:string)  [unwired: 1 in]
            n92 = call "Set All Controls Description.vi"("Description"=w276, "VI Ref"=w278) -> ()  [unwired: 9 in, 1 out]
            n93 = call "AlliGator Batch Export Status.vi"("Set/Get (F)"=TRUE, "Conversion Jobs in"=w283) -> ("error out"=w280:errorcluster)  [unwired: 8 in, 1 out]
            n94 = property on="Conversion Jobs" class="Arr"("Value"=w283) -> ()  [unwired: 2 in, 2 out]
          }
          frame "Export Files to HDF5", "Export Files to TIFF Series" {
            w287 = 5 ("index")
            n95 = call "AlliGator Batch Export Status.vi"("Set/Get (F)"=FALSE) -> ("error out"=w301:errorcluster, "Conversion Jobs out"=w293:T21[])  [unwired: 9 in]
            n96 = for {
              tunnel: w293 -> [w325] mode=indexing
              tunnel: [w322] -> w299 if=w323
              tunnel: [w323] -> _ mode=indexing
              tunnel: [w323] -> w300
              stop <- w324 continue-if-true
              n97 = Unbundle By Name(w325) -> ("File Path"=w322:path, "Saved"=w324:bool)
              n98 = Not(x=w324) -> (.not. x?=w323:bool)
            }
            n99 = Index Array(array=w288, index=w287) -> (element=w286:string)
            n100 = call "Set All Controls Description.vi"("Description"=w286, "VI Ref"=w285) -> ()  [unwired: 9 in, 1 out]
            n101 = Empty String/Path?(string/path=w299) -> (empty?=w297:bool)
            n102 = Compound Arithmetic op=AND(invert w297, w300) -> (w298:bool)
            n103 = case shown="True" w298 {
              tunnel: w299 -> [_ w321]
              tunnel: w301 -> [w304 w309]
              tunnel: w296 -> [_ w320]
              tunnel: w295 -> [_ w319]
              tunnel: [w304 w306] -> w294
              tunnel: w293 -> [_ w313]
              tunnel: w292 -> [_ w312]
              tunnel: [w303 w310] -> w291
              tunnel: w290 -> [w303 _]
              tunnel: [_ w305] -> w289
              frame False {
                # "all files converted or no files"
              }
              frame True {
                # "Not converted & not empty"
                n104 = call "Show Animated Busy Icon with Message and Abort Button.vi"("Message"=w312, "Error In"=w309) -> ("Error Out"=w308:errorcluster)  [unwired: 17 in]
                n105 = Array Size(array=w313) -> (size(s)=w314:i32)
                n106 = call "Current Date & Time String (High Precision).vi"("Error In"=w308) -> ("Error Out"=w318:errorcluster, "time string"=w317:string, "date string"=w315:string)  [unwired: 7 in, 1 out]
                n107 = call <vilib>:"Search and Replace Pattern.vi"("string"=w312, "regular expression (\"\")"="Export Files to " ("regular expression (\"\")")) -> ("result string"=w310:string)  [unwired: 3 in, 1 out]
                n108 = Format Into String(format string="Batch Dataset File Conversion of %d files started on %s at %s", error in=w318, w314, w315, w317) -> (resulting string=w305:string, error out=w307:errorcluster)  [unwired: 1 in]
                n109 = call "AlliGator Script_Convert FLI Dataset to HDF5 or TIFF Series.vi"("Dataset Saving Options"=w319, "Dataset Loading Options"=w320, "Error In"=w307, "Destination File Type"=w310, "File Path"=w321) -> ("Error Out"=w306:errorcluster)  [unwired: 6 in]
              }
            }
          }
          frame "Close" {
            n110 = Index Array(array=w328) -> (element=w327:string)  [unwired: 1 in]
            n111 = call "Set All Controls Description.vi"("Description"=w327, "VI Ref"=w326) -> ()  [unwired: 9 in, 1 out]
            n112 = xnode "Error Ring"() -> ("error out"=w329:errorcluster)
          }
        }
      }
      event Menu Activation? {
        n113 = event-data() -> ("MenuRef"=w349:refnum<k9>)  [unwired: 1 in]
        n114 = call "Alligator Variables Storage.vi"("AlliGator Variable"=AlliGator_Variables_List."Files:Show Batch Export Help Balloons" ("Alligator Variable")) -> ("Error Out"=w339:errorcluster, "Data out"=w340:variant)  [unwired: 8 in, 1 out]
        n115 = call "Alligator Variables Storage.vi"("AlliGator Variable"=AlliGator_Variables_List."Files:Export Dataset Frames as Individual Files" ("Alligator Variable")) -> ("Error Out"=w344:errorcluster, "Data out"=w346:variant)  [unwired: 8 in, 1 out]
        n116 = call-poly "Variant to Data.vi"("Variant"=w340) -> ("Value"=w338:bool)  [unwired: 8 in]
        n117 = call-poly "Variant to Data.vi"("Variant"=w346) -> ("Value"=w345:bool)  [unwired: 8 in]
        n118 = Set Menu Item Info(6:w345, 7:"Export .ptu Frames as Individual Files" ("item tag"), 8:w344, 11:w349) -> (3:w342:refnum<k9>)  [unwired: 3 in, 1 out]
        n119 = Set Menu Item Info(6:w338, 7:"Show Help" ("item tag"), 8:w339, 11:w342) -> ()  [unwired: 3 in, 2 out]
        n120 = event-data() -> ()  [unwired: 2 in, 1 out]
      }
      event "Abort": Value Change {
        n121 = event-data() -> ()  [unwired: 1 in, 1 out]
        n122 = call "Hide Animated Busy Icon with Message and Abort Button.vi"("Message"="Conversion aborted.", "Error In"=errorcluster {"status"=FALSE, "code"=0, "source"=""}) -> ("Error Out"=w359:errorcluster)  [unwired: 17 in]
        n123 = call "Current Date & Time String (High Precision).vi"() -> ("time string"=w355:string, "date string"=w356:string)  [unwired: 8 in, 2 out]
        n124 = Format Into String(format string="Conversion aborted on %s at %s" ("Message"), error in=w359, w356, w355) -> (resulting string=w354:string, error out=w360:errorcluster)  [unwired: 1 in]
      }
    }
    n125 = call "Send Message to Notebook.vi"("Error In"=w25, "Message"=w26, "Notebook Queue"=w28) -> ("Error Out"=w24:errorcluster, "Notebook Queue"=w27:refnum<queue>)  [unwired: 5 in]
    n126 = call "Message Style.vi"() -> ()  [unwired: 1 out]
    n127 = call "Send Error to Notebook.vi"("error in (no error)"=w24, "Notebook Q"=w27) -> ()  [unwired: 9 in, 1 out]
  }
  n128 = call "Alligator Variables Storage.vi"("Get(F)/Set"=w1, "AlliGator Variable"=AlliGator_Variables_List."Files:Frames in Dataset" ("Alligator Variable"), "Data in"=w8) -> ("Error Out"=w10:errorcluster)  [unwired: 6 in, 2 out]
  n129 = call "Alligator Variables Storage.vi"("Get(F)/Set"=w1, "AlliGator Variable"=AlliGator_Variables_List."Files:Current Frame in Dataset" ("Alligator Variable"), "Error In"=w10, "Data in"=w8) -> ("Error Out"=w7:errorcluster)  [unwired: 5 in, 2 out]
  n130 = call "Alligator Variables Storage.vi"("Get(F)/Set"=w1, "AlliGator Variable"=AlliGator_Variables_List."Files:Current Frame Timestamp" ("Alligator Variable"), "Error In"=w7, "Data in"=nan) -> ("Error Out"=w4:errorcluster)  [unwired: 5 in, 2 out]
  n131 = property on="Conversion Jobs" class="Arr"(error in=w4, "Value"=w19) -> (error out=w15:errorcluster)  [unwired: 1 in, 1 out]
  n132 = invoke class="VI" method="FP.Close"(error in=w15) -> (reference out=w13:refnum<vi>, error out=w12:errorcluster)  [unwired: 2 in, 1 out]
  n133 = Close Reference(reference=w13, error in (no error)=w12) -> ()  [unwired: 1 out]
  "Message" <- ""
